vi "Log Error.vi"(8 "error in (no error)":errorcluster, 11 "Error Handler in":refnum<class "Error Handler.lvclass">) -> (0 "error out":errorcluster, 3 "Error Handler out":refnum<class "Error Handler.lvclass">)   [LabVIEW 2021, in "Error Handler.lvlib" / "Error Handler.lvclass"]
uses:
  Error Handler.lvclass
panel:
  in  "error from external source":errorcluster
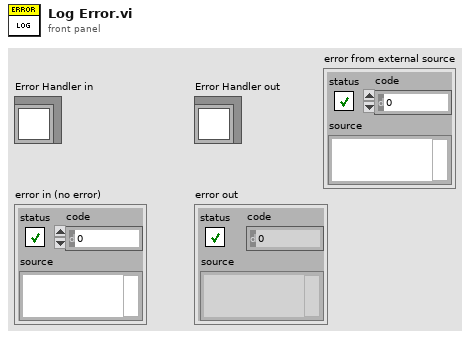
[diagram p1: front panel]
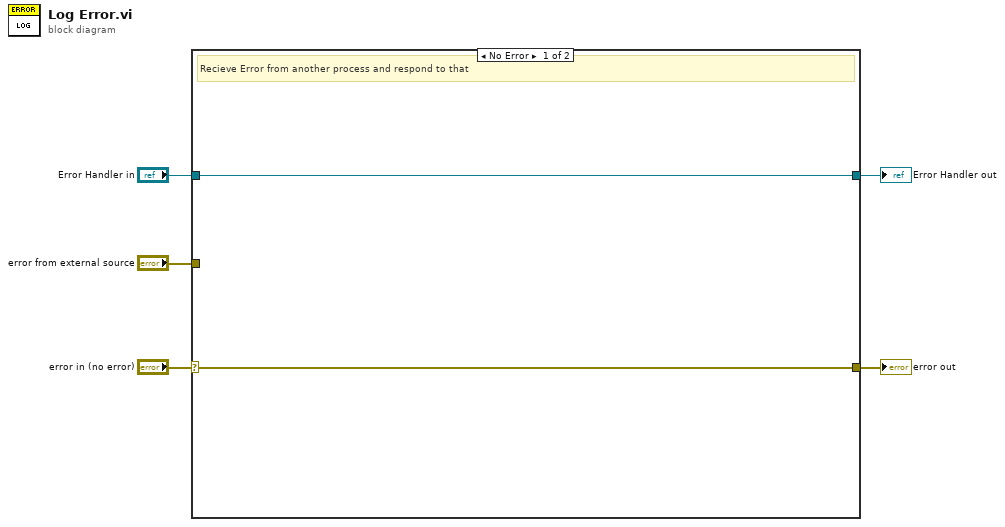
[diagram p0: block diagram]
diagram:
  n1 = case shown="No Error" "error in (no error)" {
    selector: "error in (no error)" -> [w6 w9]
    tunnel: [w6 w9] -> w4
    tunnel: [w7 w8] -> w2
    tunnel: "Error Handler in" -> [w7 w8]
    tunnel: "error from external source" -> [_ _]
    frame No Error {
      # "Recieve Error from another process and respond to that"
    }
    frame Error {
    }
  }
  "error out" <- w4
  "Error Handler out" <- w2
